vi "Calibration Applier.vi"(2 "Cal Coefficients":dbl[][](array[numeric]), 7 "Data In":dbl[](array[numeric])) -> (8 "Data Out":dbl[](array[numeric]))   [LabVIEW 2019]
uses:
  <vilib>/ptbypt/NI_PtbyPt.lvlib
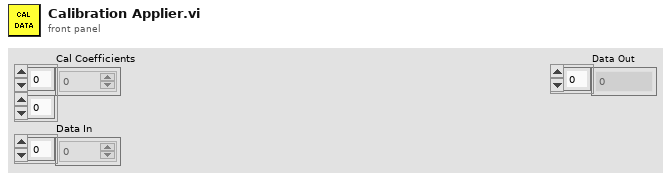
[diagram p1: front panel]
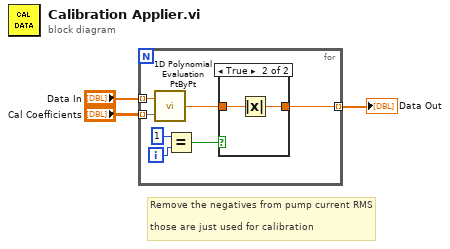
[diagram p0: block diagram]
diagram:
  # "Remove the negatives from pump current RMS\n\nthose are just used for calibration"
  n1 = for {
    tunnel: "Cal Coefficients" -> [w10] mode=indexing
    tunnel: "Data In" -> [w9] mode=indexing
    tunnel: [w5] -> w1 mode=indexing
    i -> [w8]
    n2 = call <vilib>:"1D Polynomial Evaluation PtByPt.vi"("Coefficients: a"=w10, "x"=w9) -> ("y"=w6:dbl)
    n3 = Equal?(x=1, y=w8) -> (x = y?=w4:bool)
    n4 = case shown="True" w4 {
      tunnel: w6 -> [w11 w13]
      tunnel: [w11 w12] -> w5
      frame False {
      }
      frame True {
        n5 = Absolute Value(x=w13) -> (abs(x)=w12:dbl)
      }
    }
  }
  "Data Out" <- w1
